vi "JA_Set.vi"(8 "error in (no error)":errorcluster, 9 "Jog Mode":T1 items=["-666 steps/s"=-4, "-1700 steps/s"=-3, "-100 steps/s"=-2, "-5 steps/s"=-1, "No move"=0, "+5 steps/s"=1, "+100 steps/s"=2, "+1700 steps/s"=3, "+666 steps/s"=4], 10 "Axis Number":i32, 11 "Agilis in":T2) -> (0 "error out":errorcluster, 3 "Agilis out":T2)   [LabVIEW 2016, in "Drivers.lvlib" / "Agilis.lvlib"]
doc: "Starts a jog motion at a defined speed."
uses:
  Agilis.lvlib
  AgilisCmdLib Refnum.ctl
  C:/Users/MyUser/Desktop/Trace Grabber/Drivers/Agilis/AgilisCmdLib.dll
  AgilisCmdLib.dll
  Jog Mode.ctl
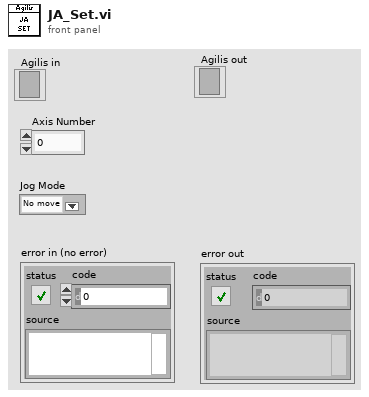
[diagram p1: front panel]
types:
  T1 = typedef "Drivers.lvlib/Agilis.lvlib/Jog Mode.ctl" = i32
  T2 = typedef "Drivers.lvlib/Agilis.lvlib/AgilisCmdLib Refnum.ctl" = refnum<k24>
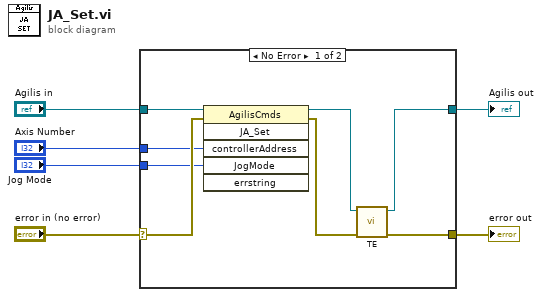
[diagram p0: block diagram]
diagram:
  n1 = case shown="No Error" "error in (no error)" {
    selector: "error in (no error)" -> [w13 w16]
    tunnel: "Agilis in" -> [w14 w15]
    tunnel: [w7 w15] -> w4
    tunnel: [w10 w16] -> w3
    tunnel: "Axis Number" -> [w12 _]
    tunnel: "Jog Mode" -> [w11 _]
    frame No Error {
      n2 = invoke class="AgilisCmds" method="JA_Set"(reference=w14, error in=w13, "controllerAddress"=w12, "JogMode"=w11) -> (reference out=w8:T2, error out=w9:errorcluster)  [unwired: 2 in, 4 out]
      n3 = call "TE.vi"("error in (no error)"=w9, "Agilis in"=w8) -> ("error out"=w10:errorcluster, "Agilis out"=w7:T2)  [unwired: 8 in]
    }
    frame Error {
    }
  }
  "Agilis out" <- w4
  "error out" <- w3
